vi "Send stimulus trigger setup.vi"(8 "error in (no error)":errorcluster, 11 "FPGA ref in":T1) -> (0 "error out":errorcluster, 3 "FPGA ref out":T1)   [LabVIEW 2013]
uses:
  RIG-SPECIFIC FILES/FPGA Refs/FPGA Ref.ctl
  FPGA DAQ/FPGA Typedefs/PXI Trigger Enable cluster.ctl
  Typedefs/HW config states enum.ctl
  FPGA DAQ/FPGA Typedefs/Stimulus trigger delays cluster.ctl
  <vilib>/rvi/interface/common/niFpgaWaitOnOcc.vi
  <vilib>/Utility/error.llb/Error Cluster From Error Code.vi
  <vilib>/rvi/errors/niLvFpgaAdjustHostInterfaceError.vi
  <vilib>/rvi/interface/nirviReadWriteControl/nirviReadWriteControl.xnode
  NiFpgaLv.dll
  <vilib>/rvi/interface/Simulation/niFpgaSimulationCallBeginRW.vi
panel:
  out "PXI Trig 0 (redundant)":bool
  out "Enable stimulus?":bool
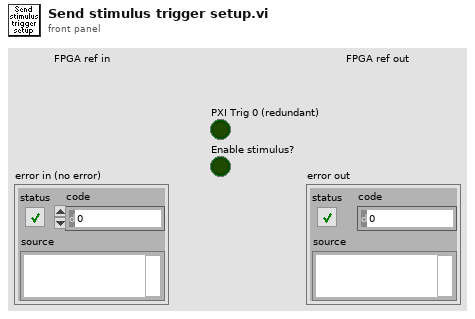
[diagram p1: front panel]
types:
  T1 = typedef "FPGA Ref.ctl" = refnum<k20>
  T2 = typedef "Stimulus trigger delays cluster.ctl" = cluster{"Trigger period in live protocols (80MHz Cycles)":u32, "Pulse width in live protocols (80MHz Cycles)":u32, "Enable stimulus in live protocols":bool, "Trigger delay in funct. protocols (80MHz Cycles)":u32, "Pulse width in funct. protocols (80MHz Cycles)":u32, "Enable stimulus in funct. protocols":bool}
  T3 = typedef "HW config states enum.ctl" = enum16{"Load from file", "Save to file", "Write all", "Read all", "Write XY stage settings", "Write DAQ FPGA settings", "Write Control FPGA settings", "Write Phys Channels", "Clear", "Compare from file"}
  T4 = typedef "PXI Trigger Enable cluster.ctl" = cluster{"Enable Trigger 1":bool, "Enable Trigger 2":bool, "Enable Trigger 3":bool, "Enable Trigger 4":bool}
  T5 = typedef "Triggers output setup.ctl" = T6[]
  T6 = typedef "Trigger setup element cluster.ctl" = cluster{"Name":string, "Output?":bool, "Output terminal":tag, "PXI backplane line":tag, "Pulse width (us)":u16}
  T7 = typedef "AOL_Globals.ctl" = cluster{"Imaging Protocol":T8, "Number of POI":u16, "Number of Miniscans":u16, "Number of Trials":u16, "Number of Cycles ":u64, "# Averaged Frames":u16, "Laser power (%)":u8, "Pockels":dbl, "Acquisition Length (sec)":dbl, "Fill time (us)":dbl, "POI Dwell time (us)":dbl, "Miniscan Dwell time per pixel (us)":dbl, "PMT 1":dbl, "PMT 2":dbl, "Back Apperture":dbl, "Frame Size":T9, "Center Frequency":dbl, "Field of View":dbl, "DwellTime (us)":dbl, "Wavelength (nm)":dbl, "Zoom":dbl, "AOL Z":dbl, "AOL Mode":T10, "GridXY":dbl, "GridZ":dbl, "TriggerPeriod (sec)":dbl, "Number of Pixels in Miniscan":u16, "Experiment folder path":path, "X centre":dbl, "Y centre":dbl, "Angle (degrees)":dbl, "Plane Mode":T11, "Threshold":u16[], "Regenerate Chirps":bool, "Rectangle ROI length (pixels)":u16, "Rectangle ROI height (pixels)":u16, "AOD fill":u16, "Samples Wait after Trigger":u16, "StartUp Delay":i32, "Slip Cycle":u32, "Add Cycle":bool}
  T8 = typedef "Imaging Protocols enum.ctl" = enum16{"AOL Z-Stack", "Motor Z Stack", "Functional Acquisition", "Single Plane Acquisition", "Volume Acquisition", "Live Imaging", "Live Plane Imaging", "Live Volume Imaging"}
  T9 = typedef "Frame Size.ctl" = u16
  T10 = typedef "AOL modes.ctl" = enum16{"Raster", "Structural", "Pointing", "Mini Scan", "Alignment"}
  T11 = typedef "Plane Mode.ctl" = u16
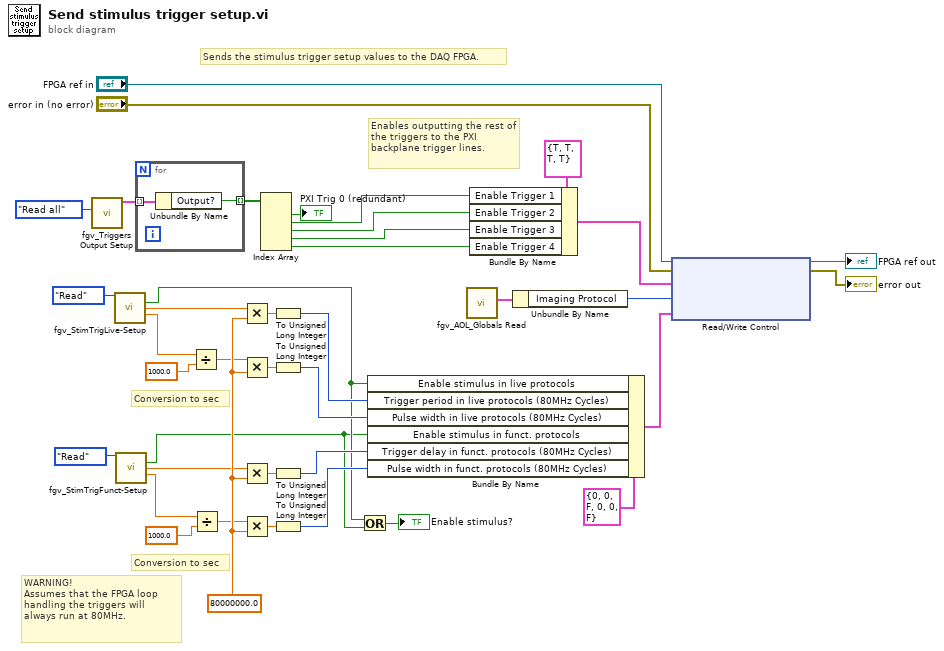
[diagram p0: block diagram]
diagram:
  w23 = 80000000.0 ("Delay in live protocols (80MHz Cycles)")
  # "Conversion to sec"
  # "Conversion to sec"
  # "WARNING!\nAssumes that the FPGA loop handling the triggers will always run at 80MHz."
  # "Enables outputting the rest of the triggers to the PXI backplane trigger lines."
  # "Sends the stimulus trigger setup values to the DAQ FPGA."
  n1 = call "fgv_Triggers Output Setup.vi"("Function"=HW_config_states_enum."Read all") -> ("Triggers output setup"=w12:T5)  [unwired: 9 in, 1 out]
  n2 = call "fgv_StimTrigLive-Setup.vi"("Function"=enum16{"Intialize", "Write", "Read", "Clear"}."Read") -> ("Live stim.trig.enable"=w18:bool, "Live stim.trig.period (sec)"=w5:dbl, "Live stim.trig.width (ms)"=w14:dbl)  [unwired: 11 in, 1 out]
  n3 = call "fgv_StimTrigFunct-Setup.vi"("Function"=enum16{"Intialize", "Write", "Read", "Clear"}."Read") -> ("Live stim.trig.enable"=w17:bool, "Funct stim.trig.delay (sec)"=w3:dbl, "Funct stim.trig.width (ms)"=w15:dbl)  [unwired: 11 in, 1 out]
  n4 = for {
    tunnel: w12 -> [w42] mode=indexing
    tunnel: [w41] -> w11 mode=indexing
    n5 = Unbundle By Name(w42) -> ("Output?"=w41:bool)
  }
  n6 = Divide(x=w14, y=1000.0) -> (x/y=w4:dbl)
  n7 = Divide(x=w15, y=1000.0) -> (x/y=w2:dbl)
  n8 = Multiply(x=w5, y=w23) -> (x*y=w32:dbl)
  n9 = Multiply(x=w4, y=w23) -> (x*y=w36:dbl)
  n10 = Multiply(x=w3, y=w23) -> (x*y=w29:dbl)
  n11 = Multiply(x=w2, y=w23) -> (x*y=w24:dbl)
  n12 = Index Array(array=w11) -> (element #1=→"PXI Trig 0 (redundant)":bool, element #2=w10:bool, element #3=w9:bool, element #4=w8:bool, element #5=w7:bool)  [unwired: 5 in]
  n13 = To Unsigned Long Integer(number=w32) -> (unsigned 32bit integer=w22:u32)
  n14 = To Unsigned Long Integer(number=w36) -> (unsigned 32bit integer=w20:u32)
  n15 = To Unsigned Long Integer(number=w29) -> (unsigned 32bit integer=w21:u32)
  n16 = To Unsigned Long Integer(number=w24) -> (unsigned 32bit integer=w19:u32)
  n17 = Or(x=w18, y=w17) -> (x .or. y?=→"Enable stimulus?":bool)
  n18 = Bundle By Name(cluster=T2 {"Trigger period in live protocols (80MHz Cycles)"=0, "Pulse width in live protocols (80MHz Cycles)"=0, "Enable stimulus in live protocols"=FALSE, "Trigger delay in funct. protocols (80MHz Cycles)"=0, "Pulse width in funct. protocols (80MHz Cycles)"=0, "Enable stimulus in funct. protocols"=FALSE} ("Trigger delays"), "Enable stimulus in live protocols"=w18, "Trigger period in live protocols (80MHz Cycles)"=w22, "Pulse width in live protocols (80MHz Cycles)"=w20, "Enable stimulus in funct. protocols"=w17, "Trigger delay in funct. protocols (80MHz Cycles)"=w21, "Pulse width in funct. protocols (80MHz Cycles)"=w19) -> (w35:T2)
  n19 = call "fgv_AOL_Globals Read.vi"() -> ("AOL_Globals"=w28:T7)  [unwired: 9 in, 2 out]
  n20 = Bundle By Name(cluster=T4 {"Enable Trigger 1"=TRUE, "Enable Trigger 2"=TRUE, "Enable Trigger 3"=TRUE, "Enable Trigger 4"=TRUE} ("PXI Backplane triggers \"Enable\" states"), "Enable Trigger 1"=w10, "Enable Trigger 2"=w9, "Enable Trigger 3"=w8, "Enable Trigger 4"=w7) -> (w33:T4)
  n21 = Unbundle By Name(w28) -> ("Imaging Protocol"=w34:T8)
  n22 = xnode ("Read/Write Control")("FPGA VI Reference In"="FPGA ref in", "error in"="error in (no error)", "PXI Trigger Enable"=w33, "Imaging Protocol"=w34, "Stimulus Trigger Setup"=w35) -> ("FPGA VI Reference Out"=→"FPGA ref out":T1, "error out"=→"error out":errorcluster)
